vi "NormalizeArray.vi"(1 "Fuel Splits":sgl[](array[numeric])) -> (0 "Normalized Fuel Splits":sgl[](array[numeric]))   [LabVIEW 2016, in "DSI-RT.lvlib"]
uses:
  DSI-RT.lvlib
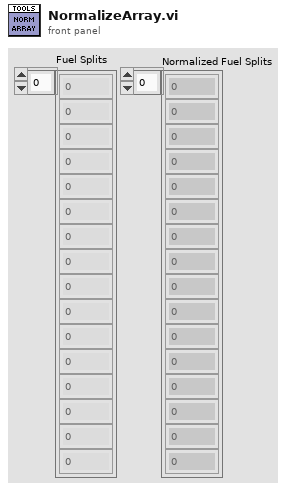
[diagram p1: front panel]
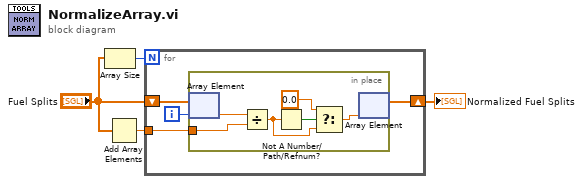
[diagram p0: block diagram]
diagram:
  n1 = Array Size(array="Fuel Splits") -> (size(s)=w2:i32)
  n2 = Add Array Elements(numeric array="Fuel Splits") -> (sum=w4:sgl)
  n3 = for {
    N: w2 -> [_]
    tunnel: w4 -> [w7]
    shift-right: [w6] -> w3
    shift-left: "Fuel Splits" -> [w8]
    i -> [w5]
    n4 = in-place {
      in-place-border: w7 -> [w13]
      n5 = in-place-array #1(w8, w5) -> (w14:sgl)
      n6 = Divide(x=w14, y=w13) -> (x/y=w11:sgl)
      n7 = Not A Number/Path/Refnum?(number/path/refnum=w11) -> (NaN/Path/Refnum?=w12:bool)
      n8 = Select(t=sgl 0.0, s=w12, f=w11) -> (s? t:f=w9:sgl)
      n9 = in-place-array #1(w9) -> (w6:sgl[])  [unwired: 1 out]
    }
  }
  "Normalized Fuel Splits" <- w3
